vi "logging.vi"() -> ()   [LabVIEW 2021]
uses:
  <vilib>/Platform/TimedLoop/XDataNode/timing_clust.ctl
  <vilib>/Platform/TimedLoop/XDataNode/nitl_modes.ctl
  <vilib>/Platform/TimedLoop/XDataNode/wakeup.ctl
  <extravilib>/ChannelInstances/Real Time Stream-i32/Instantiate.vi
  <extravilib>/ChannelInstances/Real Time Stream-i32/)Channel.vi
  <vilib>/Platform/TimedLoop/XDataNode/XDataNode.xnode
  <extravilib>/ChannelInstances/Real Time Stream-i32.lvlib
  <vilib>/Platform/TimedLoop/XDataNode/XDNodeRunTimeDep.lvlib
panel:
  in  "stop log":bool
  out "element to log":i32
  out "Logging iteration":i32
  out "logged elements":i32[](array[numeric])
  in  "stop acq":bool
  out "Acquisition iteration":i32
  in  "trigger for logging":bool=TRUE
  # "-1 represents elements not logged\nmore logic will need to be done \nfor actual clean logging"
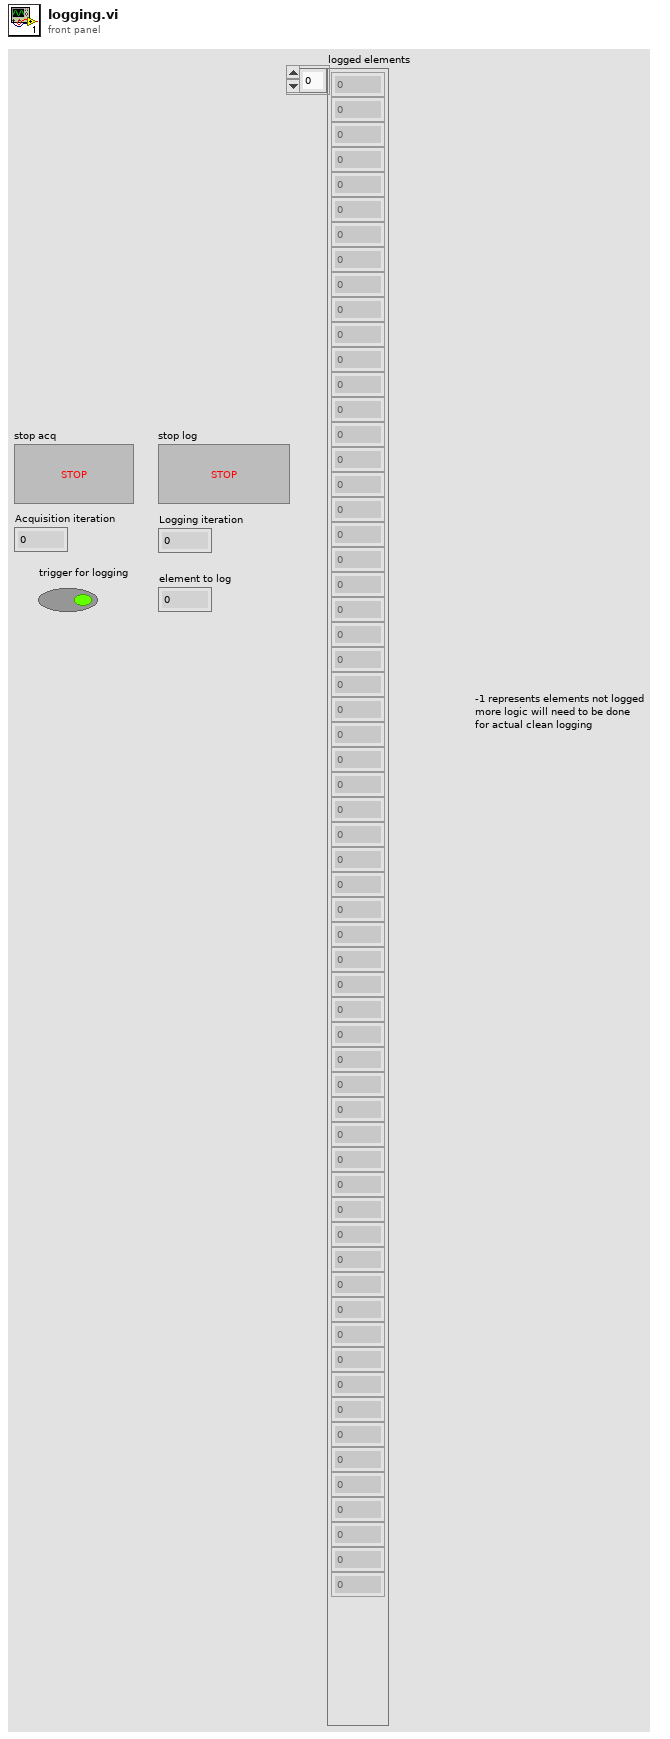
[diagram p1: front panel]
types:
  T1 = typedef "XDNodeRunTimeDep.lvlib/timing_clust.ctl" = cluster{"Expected End [f-1]":u64, "Actual End [f-1]":u64, "Finished Late? [f-1]":bool, "Expected End [i-1]":u64, "Actual End [i-1]":u64, "Finished Late? [i-1]":bool, "Expected Start [i]":u64, "Actual Start [i]":u64, "Expected Start [f]":u64, "Actual Start [f]":u64, "Source Name":string, "Structure Name":string, "Period":i64, "Deadline":i64, "Offset":i64, "Start":i64, "Priority":i32, "Timeout":i32, "Mode":T2, "Wakeup Reason":T3, "Error":errorcluster, "Source Type":string, "Secondary Source Type":string, "Global End Time":u64, "Global Start Time":u64, "Frame Duration":u64, "Iteration Duration":u64, "Assigned CPU":i32, "I/O Scan Engine Mode":u32}
  T2 = typedef "XDNodeRunTimeDep.lvlib/nitl_modes.ctl" = enum32{"No Change", "Process missed periods, maintain original phase", "Discard missed periods, maintain original phase", "Process missed periods, ignore original phase", "Discard missed periods, ignore original phase"}
  T3 = typedef "XDNodeRunTimeDep.lvlib/wakeup.ctl" = enum32{"Normal", "Aborted", "Asynchronous wakeup", "Timing source error", "Timed loop error", "Timeout"}
  T4 = typedef "Real Time Stream-i32.lvlib/)Channel.ctl" = refnum<queue>
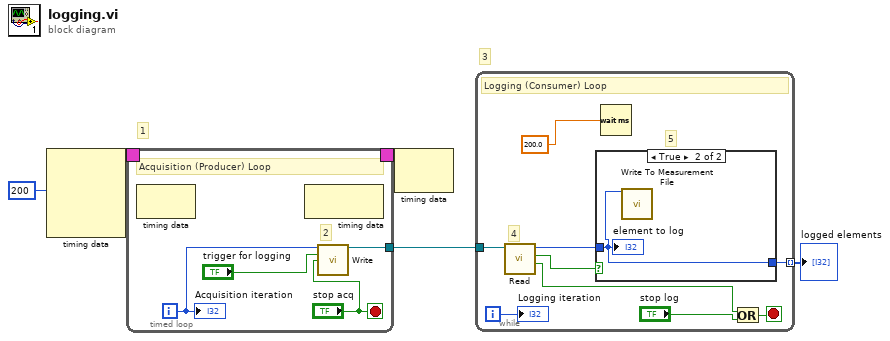
[diagram p0: block diagram]
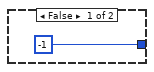
[diagram p2: hidden frame]
diagram:
  # "3"
  # "1"
  n1 = node-c288(i64 200 ("Period")) -> (w5:T1)  [unwired: 3 in]
  n2 = timed-loop {
    tunnel: [w8] -> w1
    timing: w5 -> [_]
    timing-out: [_] -> w4
    i -> [w9]
    stop <- "stop acq" stop-if-true
    # "2"
    # "Acquisition (Producer) Loop"
    n3 = node-c288() -> ()  [unwired: 1 in, 1 out]
    n4 = node-c288() -> ()  [unwired: 1 in, 1 out]
    n5 = call <extravilib>:"Write.vi"("element"=w9, "element valid? (T)"="trigger for logging", "last element? (F)"="stop acq") -> ("channel"=w8:T4)  [unwired: 10 in, 2 out]
    "Acquisition iteration" <- w9
  }
  n6 = node-c288(w4) -> ()  [unwired: 1 out]
  n7 = while {
    tunnel: w1 -> [w20]
    tunnel: [w16] -> w2 mode=indexing
    i -> [w17]
    stop <- w15 stop-if-true
    # "5"
    # "4"
    # "Logging (Consumer) Loop"
    n8 = call <extravilib>:"Read.vi"("channel"=w20) -> ("done?"=w13:bool, "element valid?"=w19:bool, "element"=w18:i32)  [unwired: 6 in, 2 out]
    n9 = case shown="True" w19 {
      tunnel: w18 -> [_ w22]
      tunnel: [-1 ("element") w22] -> w16
      frame False {
      }
      frame True {
        n10 = call "Write To Measurement File"("Signals"=w22) -> ()  [unwired: 16 in, 3 out]
        "element to log" <- w22
      }
    }
    n11 = Wait (ms)(milliseconds to wait=200.0 ("y")) -> ()  [unwired: 1 out]
    n12 = Or(x=w13, y="stop log") -> (x .or. y?=w15:bool)
    "Logging iteration" <- w17
  }
  "logged elements" <- w2
